vi "DataProcess_Tension.vi"() -> ()   [LabVIEW 2016]
uses:
  <vilib>/Utility/file.llb/Write Delimited Spreadsheet (DBL).vi
  <vilib>/AuZn/auzn custom VIs/AuZnCustomVI.lvlib
panel:
  in  "Output Path":path
  out "Total":i32
  out "Current":i32
  in  "pattern":string
  in  "Path":path
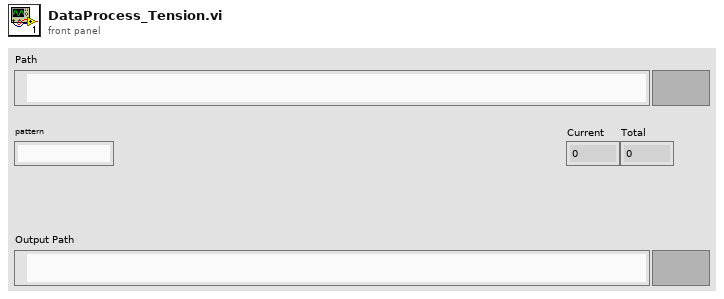
[diagram p1: front panel]
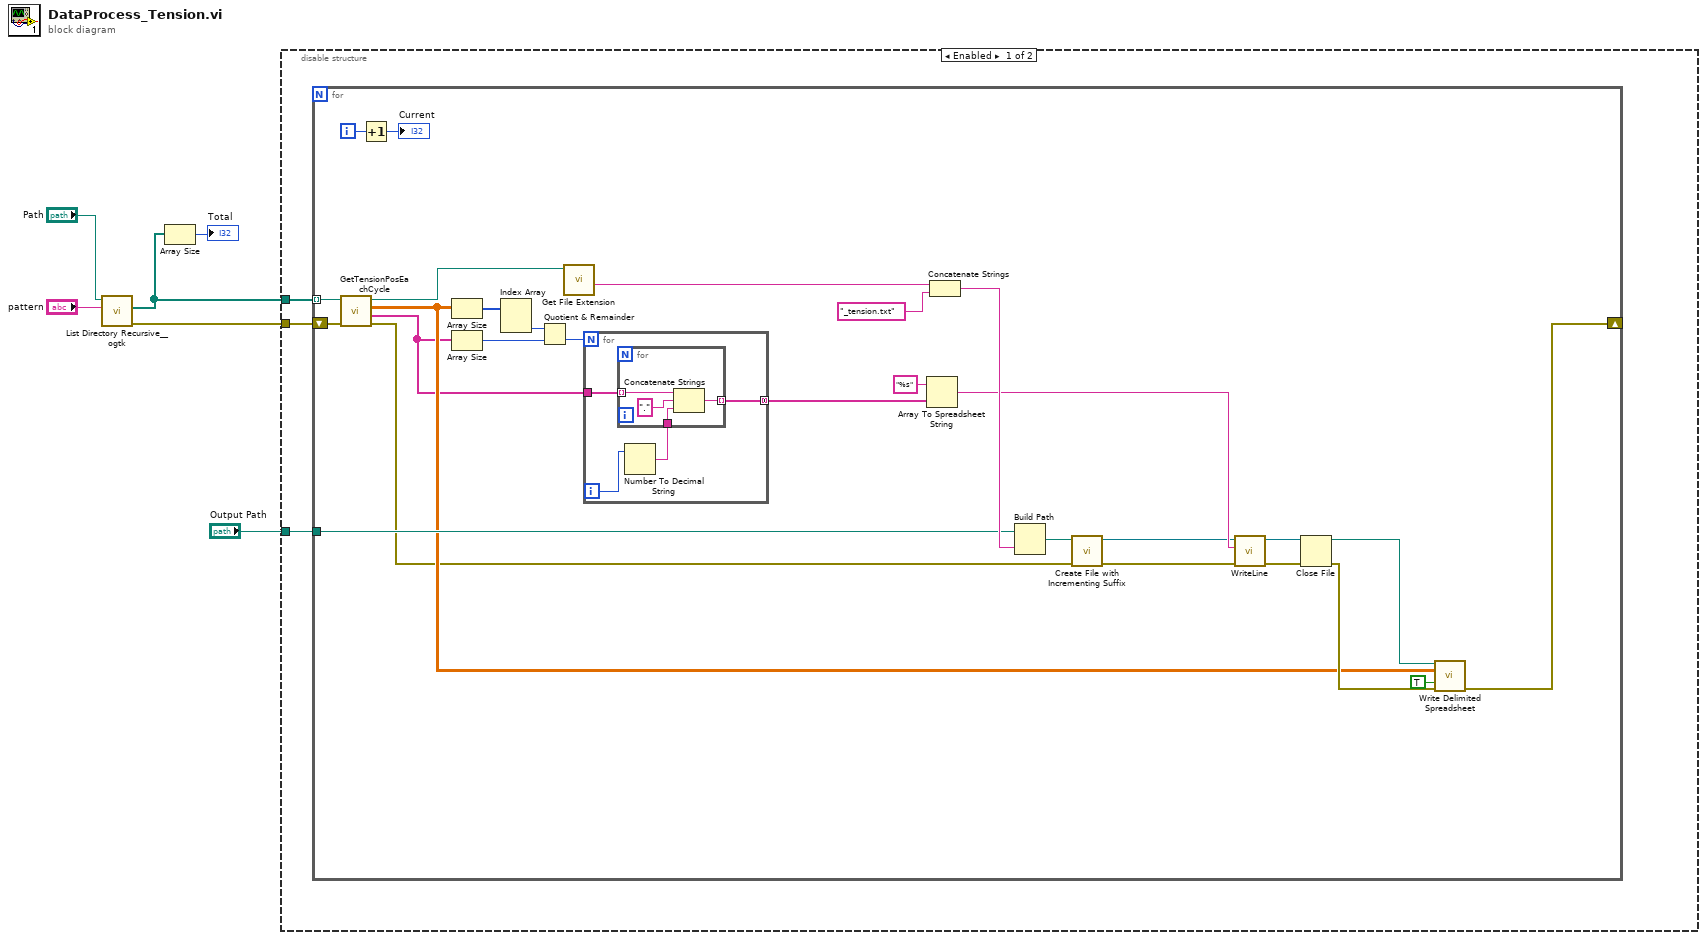
[diagram p0: block diagram]
diagram:
  n1 = call <userlib>:"List Directory Recursive__ogtk.vi"("pattern"="pattern", "Path"="Path") -> ("error out"=w1:errorcluster, "file paths"=w4:path[])  [unwired: 6 in, 2 out]
  n2 = Array Size(array=w4) -> (size(s)=→"Total":i32)
  n3 = disable-structure shown="Enabled" {
    disable-tunnel: w4 -> [w9 _]
    disable-tunnel: "Output Path" -> [w8 _]
    disable-tunnel: w1 -> [w7 _]
    frame Enabled {
      n4 = for {
        tunnel: w9 -> [w15] mode=indexing
        tunnel: w8 -> [w33]
        shift-right: [w32] -> _
        shift-left: w7 -> [w14]
        i -> [w37]
        n5 = call "GetTensionPosEachCycle.vi"("error in (no error)"=w14, "Path"=w15) -> ("error out"=w10:errorcluster, "VarColHeaders"=w11:string[], "JAEachCycle"=w12:dbl[][], "Path dup"=w13:path)  [unwired: 6 in]
        n6 = Increment(x=w37) -> (x+1=→"Current":i32)
        n7 = Array Size(array=w12) -> (size(s)=w31:i32[])
        n8 = Array Size(array=w11) -> (size(s)=w30:i32)
        n9 = Index Array(array=w31) -> (element #2=w24:i32)  [unwired: 2 in, 1 out]
        n10 = Quotient & Remainder(x=w24, y=w30) -> (floor(x/y)=w29:i32)  [unwired: 1 out]
        n11 = call <vilib>:"Get File Extension.vi"("file"=w13) -> ("filename without extension"=w25:string)  [unwired: 6 in, 4 out]
        n12 = for {
          N: w29 -> [_]
          tunnel: w11 -> [w41]
          tunnel: [w38] -> w28 mode=concatenating
          i -> [w40]
          n13 = Number To Decimal String(number=w40) -> (decimal integer string=w39:string)  [unwired: 1 in]
          n14 = for {
            tunnel: w41 -> [w45] mode=indexing
            tunnel: w39 -> [w44]
            tunnel: [w42] -> w38 mode=indexing
            n15 = Concatenate Strings(w45, "." ("string"), w44) -> (w42:string)
          }
        }
        n16 = Array To Spreadsheet String(array=w28, 3:"%s" ("format string")) -> (spreadsheet string=w26:string)  [unwired: 1 in]
        n17 = Concatenate Strings(w25, "_tension.txt" ("string")) -> (w35:string)
        n18 = Build Path(base path=w33, name or relative path=w35) -> (appended path=w18:path)
        n19 = call <vilib>:"Create File with Incrementing Suffix.vi"("error in (no error)"=w10, "file path"=w18) -> ("error out"=w16:errorcluster, "refnum out"=w17:refnum<file>)  [unwired: 7 in, 1 out]
        n20 = call <vilib>:"WriteLine.vi"("error in (no error)"=w16, "text"=w26, "refnum in"=w17) -> ("error out"=w20:errorcluster, "refnum out"=w19:refnum<file>)  [unwired: 6 in, 1 out]
        n21 = Close File(refnum=w19, error in=w20) -> (path=w23:path, error out=w22:errorcluster)
        n22 = call-poly <vilib>:"Write Delimited Spreadsheet.vi"("file path (dialog if empty)"=w23, "2D data"=w12, "append to file? (new file:F)"=TRUE ("append to file? (F)"), "error in (no error)"=w22) -> ("error out"=w32:errorcluster)  [unwired: 10 in, 1 out]
      }
    }
    frame Disabled {
    }
  }
